vi "Remove Sequencer ARB Files.vi"(8 "error in (no error)":errorcluster, 9 "Indices":i32[](array[numeric]), 10 "Instance (1)":i32=1, 11 "VISA resource name":refnum<visa-resource-name>) -> (0 "error out":errorcluster, 3 "VISA resource name out":refnum<visa-resource-name>)   [LabVIEW 2020, in "Rohde&Schwarz CMXP GPRF.lvlib"]
doc: "Removes selected files from the ARB file pool.\n\nAttribute:\nRSCMXPGPRF_ATTR_SEQUENCER_REMOVE_ARB_FILES\n\nRemote-control command:\nSOURce:GPRF:GEN<i>:SEQuencer:APOol:REMove"
uses:
  <instrlib>/Rohde&Schwarz CMXP GPRF/Rohde&Schwarz CMXP GPRF.lvlib
  <instrlib>/Rohde&Schwarz CMXP GPRF/Private/rsidr_core.llb/rsidr_core.lvlib
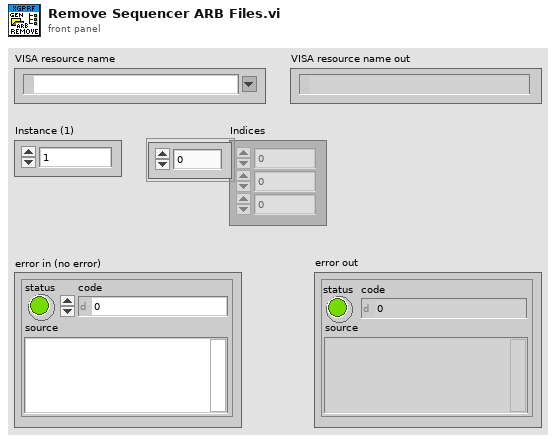
[diagram p1: front panel]
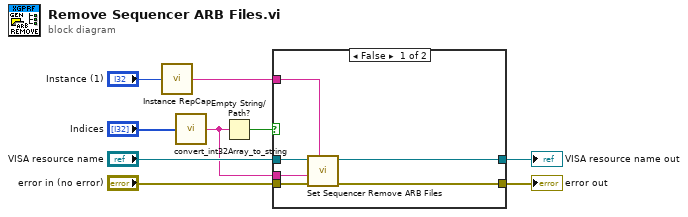
[diagram p0: block diagram]
diagram:
  n1 = call <instrlib>:"Instance RepCap.vi"("Instance in"="Instance (1)") -> ("Instance out"=w3:string)
  n2 = call <instrlib>:"convert_int32Array_to_string.vi"("I32 array in"="Indices") -> ("string out"=w2:string)  [unwired: 4 in]
  n3 = Empty String/Path?(string/path=w2) -> (empty?=w1:bool)
  n4 = case shown="False" w1 {
    tunnel: "error in (no error)" -> [w15 w16]
    tunnel: "VISA resource name" -> [w14 w17]
    tunnel: [w13 w16] -> w5
    tunnel: [w12 w17] -> w4
    tunnel: w3 -> [w11 _]
    tunnel: w2 -> [w10 _]
    frame False {
      n5 = call "Set Sequencer Remove ARB Files"("Repeated Capabilities"=w11, "error in (no error)"=w15, "Sequencer Remove ARB Files ()"=w10, "instrument handle"=w14) -> ("error out"=w13:errorcluster, "instrument handle out"=w12:refnum<visa-resource-name>)  [unwired: 6 in]
    }
    frame True {
    }
  }
  "error out" <- w5
  "VISA resource name out" <- w4
